vi "Start Cycle.vi"(8 "error in (no error)":errorcluster, 10 "Context in":refnum<class "Context.lvclass">, 11 "Idle in":refnum<class "Idle.lvclass">) -> (0 "error out":errorcluster, 2 "Context out":refnum<class "Context.lvclass">, 3 "State out":refnum<class "State.lvclass">)   [LabVIEW 2024, in "State.lvlib" / "Idle.lvclass"]
uses:
  Idle.lvclass
  Idle.lvclass/Idle.ctl
  Active/Active.lvclass
  State/State.lvclass
  C:/Users/uspoaotto/OneDrive - Oregon Tool/Desktop/working copies/stateMachineActor/src/State Machine/State/State/State.lvclass
  C:/Users/uspoaotto/OneDrive - Oregon Tool/Desktop/working copies/stateMachineActor/src/State Machine/State/~State/~State.lvclass
  C:/Users/uspoaotto/OneDrive - Oregon Tool/Desktop/working copies/stateMachineActor/src/State Machine/State/Idle/Idle.lvclass
  C:/Users/uspoaotto/OneDrive - Oregon Tool/Desktop/working copies/stateMachineActor/src/State Machine/State/Active/Active.lvclass
  Context/Context/Context.lvclass
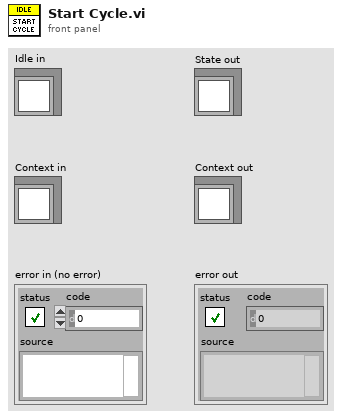
[diagram p1: front panel]
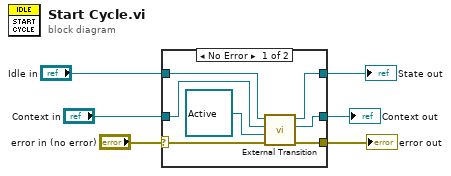
[diagram p0: block diagram]
diagram:
  n1 = case shown="No Error" "error in (no error)" {
    selector: "error in (no error)" -> [w10 w15]
    tunnel: "Idle in" -> [w13 w16]
    tunnel: [w9 w15] -> w5
    tunnel: [w7 w16] -> w3
    tunnel: "Context in" -> [w11 w14]
    tunnel: [w8 w14] -> w1
    frame No Error {
      n2 = call "External Transition.vi"("error in (no error)"=w10, "Target State"=refnum<class "Active.lvclass"> refnum ("State Machine.lvlib:State.lvlib:Active.lvclass"), "Context in"=w11, "State in"=w13) -> ("error out"=w9:errorcluster, "Context out"=w8:refnum<class "Context.lvclass">, "State out"=w7:refnum<class "State.lvclass">)  [unwired: 5 in]
    }
    frame Error {
    }
  }
  "error out" <- w5
  "State out" <- w3
  "Context out" <- w1
